vi "ISMBUS_EXAMPLE2.vi"() -> ()   [LabVIEW 2016]
uses:
  ISMBUS_Module.ctl
  ISMBUS_Channel.ctl
  ISMBUS32.DLL
panel:
  out "错误输出":errorcluster
  out "strOutput 2":string
  in  "Icp100.IActiveICP100":refnum<k7>
  out "strOutput":string
  in  "Select COM Port":i32
  in  "empty String":string
  out "ret 2":i32
  in  "ident":bool
  out "ret":i32
  in  "Listenfeld":i32(listbox)
  out "Rückgabetyp 2":i32
  in  "ConfigPfad":path
  in  "Registerkarte":T1(tab)
  out "Paramfile":string
  in  "Read PRO":bool
  in  "Write PRO":bool
  in  "Open":bool
  out "Address":i32
  out "Rückgabetyp":i32
  in  "Selected Module":T2
  in  "?":bool
  in  "ModuleArray":T2[](array[typedef])
  in  "scan":bool
  in  "select":bool
  out "Selected Modul":string
  in  "Online Modules":i32(listbox)
  out "error out":errorcluster
  in  "Fehler (Eingang, kein Fehler)":errorcluster
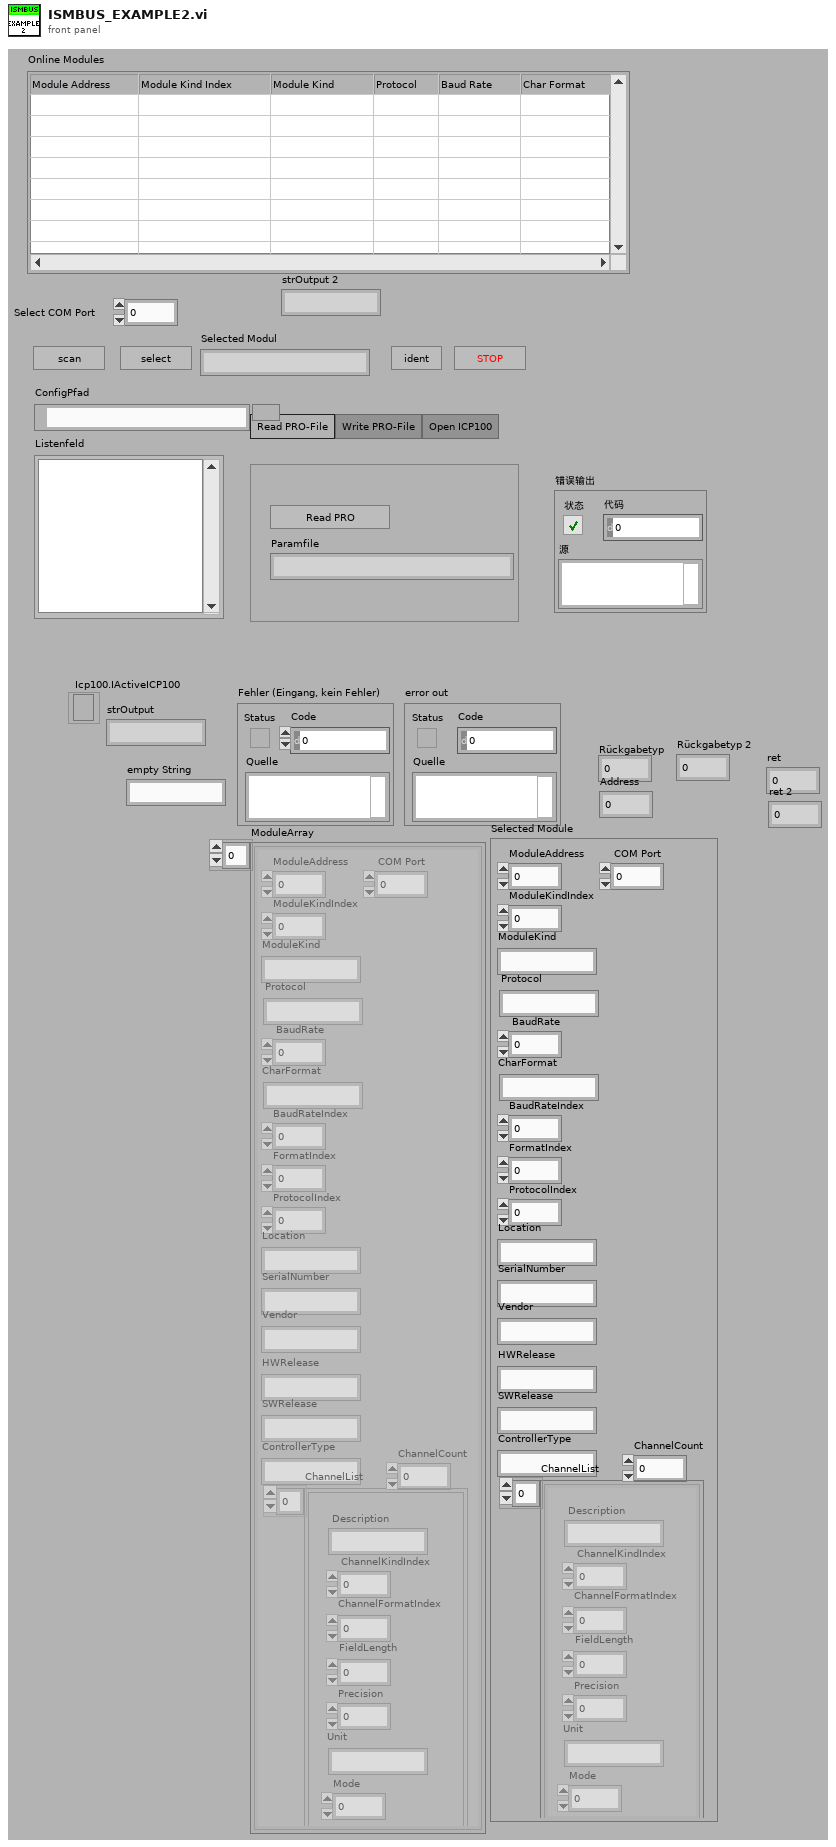
[diagram p1: front panel]
types:
  T1 = enum32{"Read PRO-File", "Write PRO-File", "Open ICP100"}
  T2 = typedef "ISMBUS_Module.ctl" = cluster{"ModuleAddress":i32, "ModuleKindIndex":i32, "ModuleKind":string, " Protocol":string, " BaudRate":i32, "CharFormat":string, "BaudRateIndex":i32, "FormatIndex":i32, "ProtocolIndex":i32, "Location":string, "SerialNumber":string, "Vendor":string, "HWRelease":string, "SWRelease":string, "ControllerType":string, "ChannelList":T3[], "ChannelCount":i32, " COM Port":i32}
  T3 = typedef "ISMBUS_Channel.ctl" = cluster{" Description":string, " ChannelKindIndex":i32, "ChannelFormatIndex":i32, " FieldLength":i32, "Precision":i32, "Unit":string, "Mode":i32}
  T4 = enum16{"idle", "scan", "select", "config", "upload", "open"}
  T5 = enum16{"idle", "scan", "select", "config", "upload"}
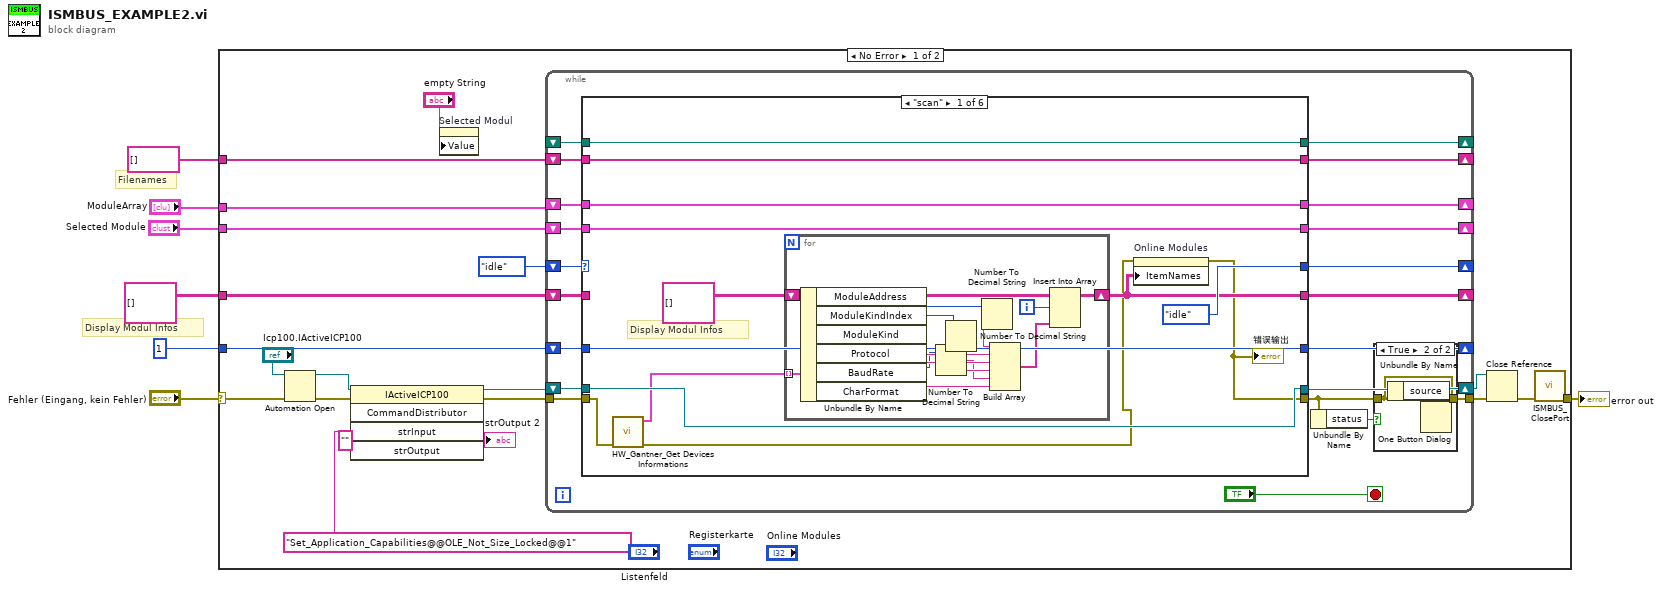
[diagram p0: block diagram]
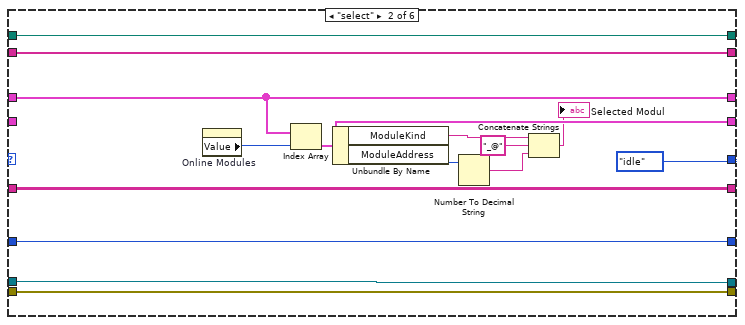
[diagram p3: hidden frame]
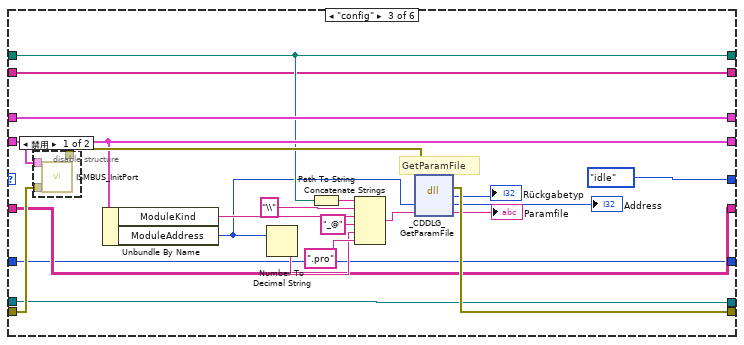
[diagram p4: hidden frame]
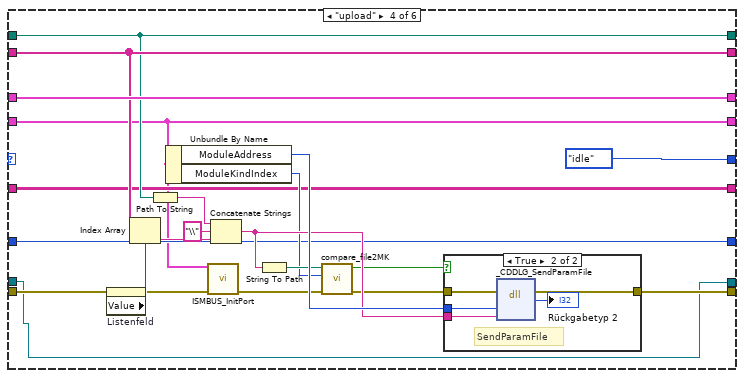
[diagram p6: hidden frame]
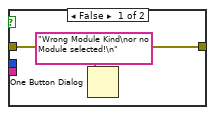
[diagram p7: hidden frame]
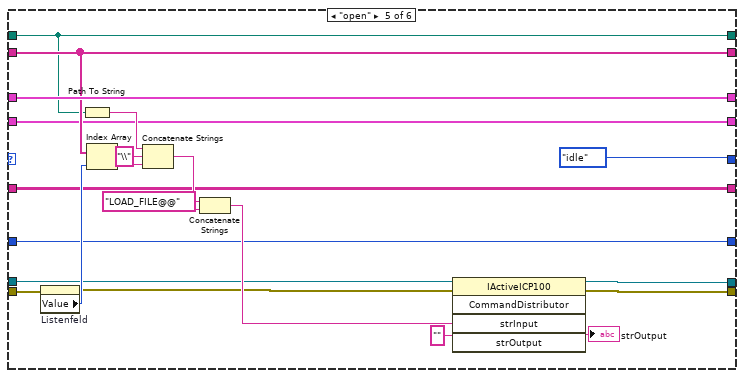
[diagram p8: hidden frame]
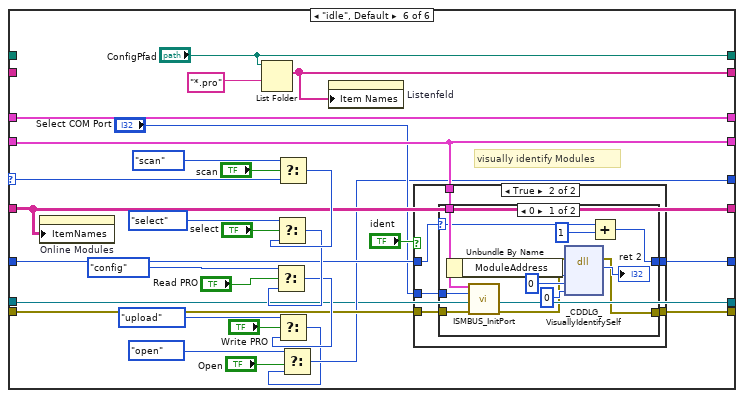
[diagram p9: hidden frame]
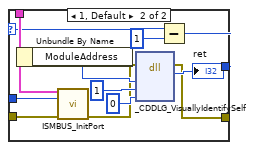
[diagram p11: hidden frame]
diagram:
  # "Display Modul Infos"
  # "Filenames"
  n1 = case shown="No Error" "Fehler (Eingang, kein Fehler)" {
    selector: "Fehler (Eingang, kein Fehler)" -> [w18 w230]
    tunnel: [w24 w230] -> w6
    tunnel: "ModuleArray" -> [w27 _]
    tunnel: "Selected Module" -> [w21 _]
    tunnel: string[] [] ("Dateinamen") -> [w25 _]
    tunnel: string[][] [] ("Objektnamen") -> [w23 _]
    tunnel: 1 -> [w22 _]
    frame No Error {
      n2 = Automation Open(error in (no error)=w18, Automation Refnum="Icp100.IActiveICP100") -> (Automation Refnum=w12:refnum<k7>, error out=w14:errorcluster)  [unwired: 2 in]
      n3 = invoke class="IActiveICP100" method="CommandDistributor"(reference=w12, error in=w14, "strInput"="Set_Application_Capabilities@@OLE_Not_Size_Locked@@1", "strOutput"="") -> (reference out=w11:refnum<k7>, error out=w13:errorcluster, "strOutput"=→"strOutput 2":string)  [unwired: 1 in, 2 out]
      n4 = property on="Selected Modul" class="Str"("Value"="empty String") -> ()  [unwired: 2 in, 2 out]
      n5 = while {
        tunnel: w13 -> [w48]
        tunnel: [w30] -> w16
        shift-right: [w46] -> _
        shift-left: w27 -> [w47]
        shift-right: [w44] -> _
        shift-left: T4."idle" -> [w45]
        shift-right: [w43] -> _
        shift-left: w21 -> [w42]
        shift-right: [w40] -> _
        shift-left: _ -> [w41]
        shift-right: [w39] -> _
        shift-left: w25 -> [w38]
        shift-right: [w36] -> _
        shift-left: w23 -> [w37]
        shift-right: [w34] -> _
        shift-left: w22 -> [w35]
        shift-right: [w29] -> w15
        shift-left: w11 -> [w28]
        stop <- "?" stop-if-true
        n6 = case shown="\"scan\"" w45 {
          selector: w45 -> [_ _ _ _ _ w196]
          tunnel: [T5."idle" T5."idle" T5."idle" T5."idle" T4."idle" w173] -> w44
          tunnel: w47 -> [w52 w92 w114 w140 w168 w182]
          tunnel: [w52 w92 w114 w140 w168 w182] -> w46
          tunnel: w48 -> [w55 w90 w113 w138 w163 w181]
          tunnel: [w54 w90 w111 w130 w151 w180] -> w31
          tunnel: [w57 w89 w106 w120 w154 w176] -> w43
          tunnel: w42 -> [w57 _ w106 w120 w154 w176]
          tunnel: w41 -> [w63 w88 w102 w135 w155 _]
          tunnel: [w63 w88 w102 w135 w155 "ConfigPfad"] -> w40
          tunnel: [w62 w87 w101 w136 w167 w184] -> w39
          tunnel: w38 -> [w62 w87 w101 w136 w167 _]
          tunnel: w37 -> [_ w80 w95 w124 w156 w179]
          tunnel: [w56 w80 w95 w124 w156 w179] -> w36
          tunnel: w35 -> [w59 w79 w94 w123 w153 w178]
          tunnel: [w59 w79 w94 w123 w153 w177] -> w34
          tunnel: [w58 w78 w93 w119 w150 w169] -> w29
          tunnel: w28 -> [w58 w78 w93 w119 w149 w169]
          frame "scan" {
            # "Display Modul Infos"
            n7 = call "HW_Gantner_Get Devices Informations.vi"("错误输入"=w55) -> ("错误输出"=w54:errorcluster, "ModuleArray"=w53:T2[])  [unwired: 9 in]
            "错误输出" <- w54
            n8 = for {
              tunnel: w53 -> [w74] mode=indexing
              shift-right: [w75] -> w56
              shift-left: string[][] [] ("Objektnamen") -> [w64]
              i -> [w77]
              n9 = Unbundle By Name(w74) -> ("ModuleAddress"=w73:i32, "ModuleKindIndex"=w70:i32, "ModuleKind"=w71:string, "Protocol"=w68:string, "BaudRate"=w67:i32, "CharFormat"=w65:string)
              n10 = Number To Decimal String(number=w67) -> (decimal integer string=w66:string)  [unwired: 1 in]
              n11 = Number To Decimal String(number=w70) -> (decimal integer string=w69:string)  [unwired: 1 in]
              n12 = Number To Decimal String(number=w73) -> (decimal integer string=w72:string)  [unwired: 1 in]
              n13 = Build Array(w72, w69, w71, w68, w66, w65) -> (w76:string[])
              n14 = Insert Into Array(array=w64, index (row)=w77, new element=w76) -> (w75:string[][])  [unwired: 1 in]
            }
            n15 = property on="Online Modules" class="MCListbox (strict)"("ItemNames"=w56) -> ()  [unwired: 2 in, 2 out]
          }
          frame "select" {
            n16 = property on="Online Modules" class="MCListbox (strict)"() -> ("Value"=w91:i32)  [unwired: 2 in, 2 out]
            n17 = Index Array(array=w92, index=w91) -> (element=w89:T2)
            n18 = Unbundle By Name(w89) -> ("ModuleKind"=w85:string, "ModuleAddress"=w86:i32)
            n19 = Number To Decimal String(number=w86) -> (decimal integer string=w83:string)  [unwired: 1 in]
            n20 = Concatenate Strings(w85, "_@" ("String"), w83) -> (→"Selected Modul":string)
          }
          frame "config" {
            # "GetParamFile"
            n21 = disable-structure shown="禁用" {
              disable-tunnel: w113 -> [w117 w118]
              disable-tunnel: [w116 w118] -> w112
              disable-tunnel: w106 -> [w115 _]
              frame Disabled {
                n22 = call "ISMBUS_InitPort.vi"("Module"=w115, "Fehler (Eingang - kein Fehler)"=w117) -> ("Fehler (Ausgang)"=w116:errorcluster)  [unwired: 13 in]
              }
              frame Enabled {
              }
            }
            n23 = Unbundle By Name(w106) -> ("ModuleKind"=w104:string, "ModuleAddress"=w97:i32)
            n24 = Number To Decimal String(number=w97) -> (decimal integer string=w98:string)  [unwired: 1 in]
            n25 = Path To String(path=w102) -> (string=w107:string)
            n26 = Concatenate Strings(w107, "\\" ("String"), w104, "_@" ("String"), w98, ".pro" ("String")) -> (w105:string)
            n27 = dll-call lib="ISMBUS32.DLL" fn="_CDDLG_GetParamFile"(error in=w112, "Address"=w97, "Paramfile"=w105) -> (error out=w111:errorcluster, "Rückgabetyp"=→"Rückgabetyp":i32, "Address"=→"Address":i32, "Paramfile"=→"Paramfile":string)  [unwired: 2 in, 1 out]
          }
          frame "upload" {
            n28 = property on="Listenfeld" class="LstBox (strict)"(error in=w138) -> (error out=w122:errorcluster, "Value"=w137:i32)  [unwired: 1 in, 1 out]
            n29 = Index Array(array=w136, index=w137) -> (element=w132:string)
            n30 = Path To String(path=w135) -> (string=w134:string)
            n31 = Unbundle By Name(w120) -> ("ModuleAddress"=w131:i32, "ModuleKindIndex"=w126:i32)
            n32 = call "ISMBUS_InitPort.vi"("Module"=w120, "Fehler (Eingang - kein Fehler)"=w122) -> ("Fehler (Ausgang)"=w121:errorcluster)  [unwired: 13 in]
            n33 = Concatenate Strings(w134, "\\" ("String"), w132) -> (w129:string)
            n34 = String To Path(string=w129) -> (path=w127:path)
            n35 = call "compare_file2MK.vi"("Fehler (Eingang, kein Fehler)"=w121, "ModuleKindIndex"=w126, "Pfad"=w127) -> ("error out"=w128:errorcluster, "file=module"=w125:bool)  [unwired: 7 in]
            n36 = case shown="True" w125 {
              tunnel: w131 -> [_ w147]
              tunnel: [w142 w145] -> w130
              tunnel: w129 -> [_ w144]
              tunnel: w128 -> [w142 w143]
              frame False {
                n37 = One Button Dialog(message="Wrong Module Kind\nor no Module selected!\n" ("Nachricht")) -> ()  [unwired: 1 in, 1 out]
              }
              frame True {
                # "SendParamFile"
                n38 = dll-call lib="ISMBUS32.DLL" fn="_CDDLG_SendParamFile"(error in=w143, "Address"=w147, "Paramfile"=w144) -> (error out=w145:errorcluster, "Rückgabetyp"=→"Rückgabetyp 2":i32)  [unwired: 4 in, 1 out]
              }
            }
          }
          frame "open" {
            n39 = property on="Listenfeld" class="LstBox (strict)"(error in=w163) -> (error out=w148:errorcluster, "Value"=w162:i32)  [unwired: 1 in, 1 out]
            n40 = Path To String(path=w155) -> (string=w165:string)
            n41 = Index Array(array=w167, index=w162) -> (element=w164:string)
            n42 = Concatenate Strings(w165, "\\" ("String"), w164) -> (w159:string)
            n43 = Concatenate Strings("LOAD_FILE@@" ("String"), w159) -> (w158:string)
            n44 = invoke class="IActiveICP100" method="CommandDistributor"(reference=w149, error in=w148, "strInput"=w158, "strOutput"="") -> (reference out=w150:refnum<k7>, error out=w151:errorcluster, "strOutput"=→"strOutput":string)  [unwired: 1 in, 2 out]
          }
          frame "idle", Default {
            # "visually identify Modules"
            n45 = property on="Online Modules" class="MCListbox (strict)"("ItemNames"=w179) -> ()  [unwired: 2 in, 2 out]
            n46 = List Folder(path="ConfigPfad", pattern="*.pro" ("Muster")) -> (filenames=w184:string[])  [unwired: 2 in, 3 out]
            n47 = Select(t=enum16{"idle", "scan", "select", "config"}."scan", s="scan", f=w196) -> (s? t:f=w194:T4)
            n48 = Select(t=enum16{"idle", "scan", "select", "config"}."select", s="select", f=w194) -> (s? t:f=w189:T4)
            n49 = Select(t=enum16{"idle", "scan", "select", "config"}."config", s="Read PRO", f=w189) -> (s? t:f=w186:T4)
            n50 = Select(t=T5."upload", s="Write PRO", f=w186) -> (s? t:f=w172:T4)
            n51 = Select(t=T4."open", s="Open", f=w172) -> (s? t:f=w173:T4)
            n52 = property on="Listenfeld" class="LstBox (strict)"("Item Names"=w184) -> ()  [unwired: 2 in, 2 out]
            n53 = case shown="True" "ident" {
              tunnel: w181 -> [w198 w204]
              tunnel: [w198 w205] -> w180
              tunnel: w178 -> [w199 w203]
              tunnel: [w199 w202] -> w177
              tunnel: w176 -> [_ w201]
              tunnel: "Select COM Port" -> [_ w200]
              frame False {
              }
              frame True {
                n54 = case shown="0" w203 {
                  selector: w203 -> [w206 w218]
                  tunnel: [w213 w225] -> w205
                  tunnel: w204 -> [w210 w222]
                  tunnel: [w211 w223] -> w202
                  tunnel: w201 -> [w208 w220]
                  tunnel: w200 -> [w207 w219]
                  frame 0 {
                    n55 = Unbundle By Name(w208) -> ("ModuleAddress"=w215:i32)
                    n56 = call "ISMBUS_InitPort.vi"("Module"=w208, "ComPort"=w207, "Fehler (Eingang - kein Fehler)"=w210) -> ("Fehler (Ausgang)"=w209:errorcluster)  [unwired: 12 in]
                    n57 = dll-call lib="ISMBUS32.DLL" fn="_CDDLG_VisuallyIdentifySelf"(error in=w209, "Address"=w215, "Activate"=0, "AddArgument"=0 ("bla")) -> (error out=w213:errorcluster, "Rückgabetyp"=→"ret 2":i32)  [unwired: 5 in, 1 out]
                    n58 = Add(x=w206, y=1) -> (x+y=w211:i32)
                  }
                  frame 1, Default {
                    n59 = Unbundle By Name(w220) -> ("ModuleAddress"=w227:i32)
                    n60 = call "ISMBUS_InitPort.vi"("Module"=w220, "ComPort"=w219, "Fehler (Eingang - kein Fehler)"=w222) -> ("Fehler (Ausgang)"=w221:errorcluster)  [unwired: 12 in]
                    n61 = dll-call lib="ISMBUS32.DLL" fn="_CDDLG_VisuallyIdentifySelf"(error in=w221, "Address"=w227, "Activate"=1, "AddArgument"=0 ("bla")) -> (error out=w225:errorcluster, "Rückgabetyp"=→"ret":i32)  [unwired: 5 in, 1 out]
                    n62 = Subtract(x=w218, y=1) -> (x-y=w223:i32)
                  }
                }
              }
            }
          }
        }
        n63 = Unbundle By Name(w31) -> ("status"=w32:bool)
        n64 = case shown="True" w32 {
          tunnel: w31 -> [w49 w50]
          tunnel: [w49 w50] -> w30
          frame False {
          }
          frame True {
            n65 = Unbundle By Name(w50) -> ("source"=w51:string)
            n66 = One Button Dialog(message=w51) -> ()  [unwired: 1 in, 1 out]
          }
        }
      }
      n67 = Close Reference(reference=w15, error in (no error)=w16) -> (error out=w17:errorcluster)
      n68 = call "ISMBUS_ClosePort.vi"("Fehler (Eingang - kein Fehler)"=w17) -> ("Fehler (Ausgang)"=w24:errorcluster)  [unwired: 10 in]
    }
    frame Error {
    }
  }
  "error out" <- w6
